vi "lvEtherbone.application_example_snoop.vi"() -> ()   [LabVIEW 2009, in "lvEtherbone.lvlib"]
doc: "This example demonstrate the implementation of a virtual Etherbone device.\n\nIn case of a timeout, the example writes the number of iterations to the baseAddress as an array of eight bytes. If somebody writes data to THIS virtual device, an array of eight bytes is read from (baseAddress+8)."
uses:
  lvEtherbone.lvlib
  lvEtherbone.lveb_activity_t.ctl
panel:
  out "nOfRead":i32=6
  out "nOfWrite":i32=6
  out "iterations":i32=60
  out "lastActivity":T1=enum."EBACT_TIMEDOUT"
  in  "timeout [ms]":i32=1000
  out "receivedData":u8[](array[numeric]) format="%.0x"
  out "error out":errorcluster
  in  "stop":bool
  in  "maskAddress":i32=255 format="%.0x"
  in  "baseAddress":u64=32768 format="%.0x"
  in  "port":i32=5555
  # "receivedData is read from the address \"baseaddress+8\"!"
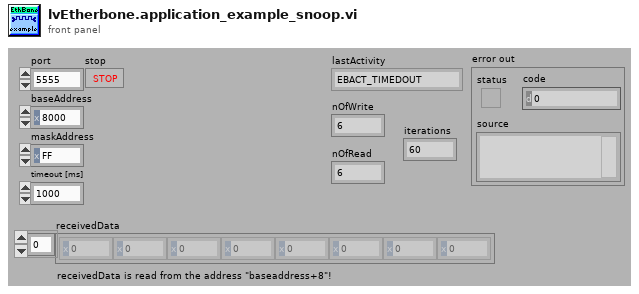
[diagram p1: front panel]
types:
  T1 = typedef "lvEtherbone.lvlib/lvEtherbone.lveb_activity_t.ctl" = enum32{"EBACT_UNKNOWN", "EBACT_TIMEDOUT", "EBACT_READ", "EBACT_WRITE", "EBACT_RW"}
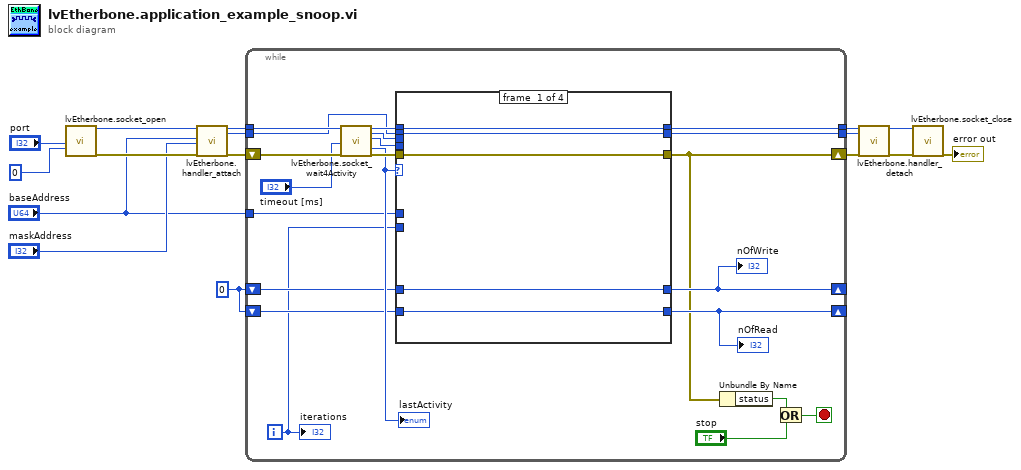
[diagram p0: block diagram]
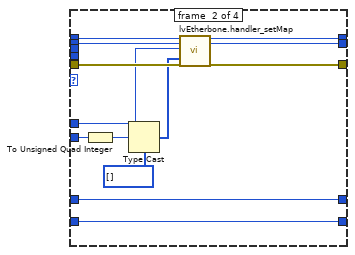
[diagram p2: hidden frame]
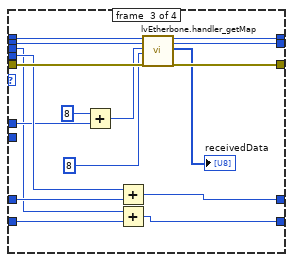
[diagram p3: hidden frame]
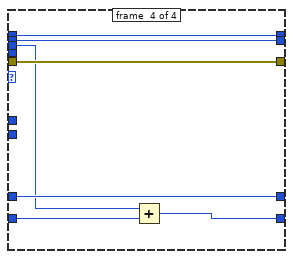
[diagram p4: hidden frame]
diagram:
  w2 = 0
  n1 = call "lvEtherbone.socket_open.vi"("port"="port", "flags"=0) -> ("eb_socket_ID"=w14:i32, "error out"=w13:errorcluster)  [unwired: 15 in, 1 out]
  n2 = call "lvEtherbone.handler_attach.vi"("eb_socket_ID"=w14, "baseAddress"="baseAddress", "maskAddress"="maskAddress", "error in (no error)"=w13) -> ("eb_socket_ID out"=w3:i32, "eb_handlerID"=w9:i32, "error out"=w7:errorcluster)  [unwired: 12 in, 1 out]
  n3 = while {
    tunnel: w3 -> [w34]
    tunnel: [w37] -> w10
    tunnel: w9 -> [w29]
    tunnel: [w36] -> w8
    shift-right: [w24] -> w6
    shift-left: w7 -> [w35]
    shift-right: [w27] -> _
    shift-left: w2 -> [w28]
    shift-right: [w25] -> _
    shift-left: w2 -> [w26]
    tunnel: "baseAddress" -> [w18]
    i -> [w17]
    stop <- w21 stop-if-true
    n4 = call "lvEtherbone.socket_wait4Activity.vi"("eb_socketID"=w34, "timeout [ms]"="timeout [ms]", "error in (no error)"=w35) -> ("eb_socketID out"=w30:i32, "nRead"=w19:i32, "nWrite"=w20:i32, "lastActivity"=w31:T1, "error out"=w32:errorcluster)  [unwired: 10 in, 2 out]
    "lastActivity" <- w31
    n5 = case shown="\"EBACT_TIMEDOUT\"" w31 {
      tunnel: [w42 w52 w72 w77] -> w24
      tunnel: [w40 w50 w71 w79] -> w37
      tunnel: [w41 w49 w70 w78] -> w36
      tunnel: w32 -> [w42 w53 w69 w77]
      tunnel: w30 -> [w40 w51 w68 w79]
      tunnel: w29 -> [w41 w48 w67 w78]
      tunnel: w28 -> [w39 w55 w66 w76]
      tunnel: [w39 w55 w65 w76] -> w27
      tunnel: w26 -> [w38 w54 w58 w75]
      tunnel: [w38 w54 w57 w74] -> w25
      tunnel: w20 -> [_ _ w64 _]
      tunnel: w19 -> [_ _ w56 w73]
      tunnel: w17 -> [_ w44 _ _]
      tunnel: w18 -> [_ w45 w61 _]
      frame #0 {
      }
      frame #1 {
        n6 = To Unsigned Quad Integer(1:w44) -> (0:w43:u64)
        n7 = Type Cast(type=u8[] [], x=w43) -> (*(type *) &x=w46:u8[])
        n8 = call "lvEtherbone.handler_setMap.vi"("eb_socketID"=w51, "eb_handlerID"=w48, "address"=w45, "data"=w46, "error in (no error)"=w53) -> ("eb_socketID out"=w50:i32, "eb_handlerID out"=w49:i32, "error out"=w52:errorcluster)  [unwired: 11 in, 1 out]
      }
      frame #2 {
        n9 = Add(x=u64 8, y=w61) -> (x+y=w62:u64)
        n10 = Add(x=w64, y=w66) -> (x+y=w65:i32)
        n11 = Add(x=w56, y=w58) -> (x+y=w57:i32)
        n12 = call "lvEtherbone.handler_getMap.vi"("eb_socket_ID"=w68, "eb_handlerID"=w67, "address"=w62, "size"=8, "error in (no error)"=w69) -> ("eb_socket_ID out"=w71:i32, "eb_handlerID out"=w70:i32, "data"=→"receivedData":u8[], "error out"=w72:errorcluster)  [unwired: 10 in, 1 out]
      }
      frame #3 {
        n13 = Add(x=w73, y=w75) -> (x+y=w74:i32)
      }
    }
    "nOfWrite" <- w27
    "nOfRead" <- w25
    n14 = Unbundle By Name(w24) -> ("status"=w23:bool)
    n15 = Or(x=w23, y="stop") -> (x .or. y?=w21:bool)
    "iterations" <- w17
  }
  n16 = call "lvEtherbone.handler_detach.vi"("eb_socketID"=w10, "eb_handlerID"=w8, "error in (no error)"=w6) -> ("eb_socketID out"=w11:i32, "error out"=w5:errorcluster)  [unwired: 14 in, 1 out]
  n17 = call "lvEtherbone.socket_close.vi"("eb_socket_ID"=w11, "error in (no error)"=w5) -> ("error out"=→"error out":errorcluster)  [unwired: 16 in, 1 out]
